vi "Gyro Angle Calibration.vi"(9 "turning joystick input":dbl, 11 "Gyro":dbl) -> (3 "adjusted turning output":dbl)   [LabVIEW 2018]
uses:
  Infrastructure/Constants.vi
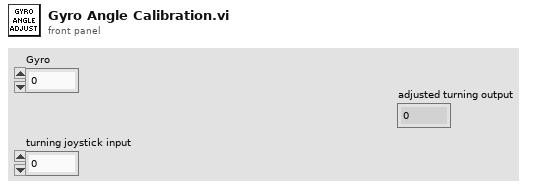
[diagram p1: front panel]
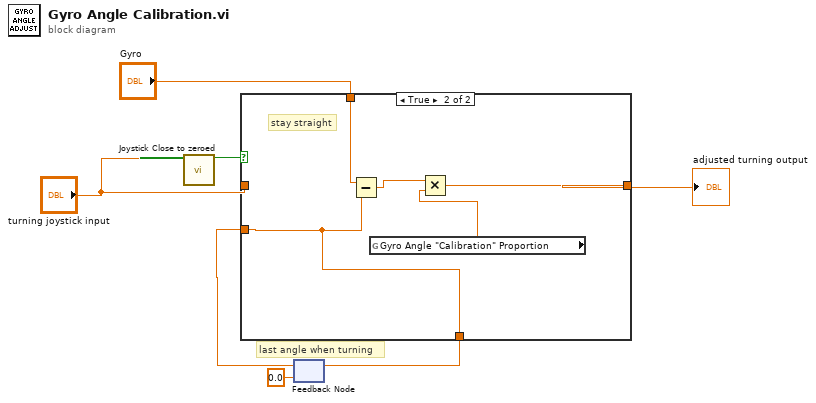
[diagram p0: block diagram]
diagram:
  # "last angle when turning"
  n1 = call "Joystick Close to zeroed.vi"("Joystick"="turning joystick input") -> ("=0?"=w7:bool)  [unwired: 10 in]
  n2 = feedback #1(0.0 ("where we are")) -> (w4:dbl)
  n3 = case shown="True" w7 {
    tunnel: "Gyro" -> [w9 w13]
    tunnel: [w9 w12] -> w5
    tunnel: w4 -> [_ w12]
    tunnel: [w8 w11] -> w1
    tunnel: "turning joystick input" -> [w8 _]
    frame False {
    }
    frame True {
      # "stay straight"
      n4 = Subtract(x=w13, y=w12) -> (x-y=w14:dbl)
      n5 = global read "Constants.vi" "Gyro Angle \"Calibration\" Proportion"() -> (w10:dbl)
      n6 = Multiply(x=w14, y=w10) -> (x*y=w11:dbl)
    }
  }
  "adjusted turning output" <- w1
  n7 = feedback-in #1(w5) -> ()
